vi "check_cancel_token.vi"(8 "error in (no error)":errorcluster) -> (0 "error out":errorcluster, 2 "exit_thread":bool)   [LabVIEW 2021, in "system.threading.lvclass"]
uses:
  system.threading.lvclass
  system.threading.lvclass/system.threading.ctl
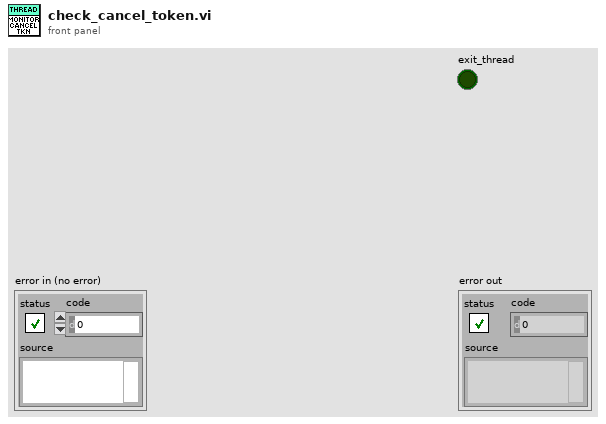
[diagram p1: front panel]
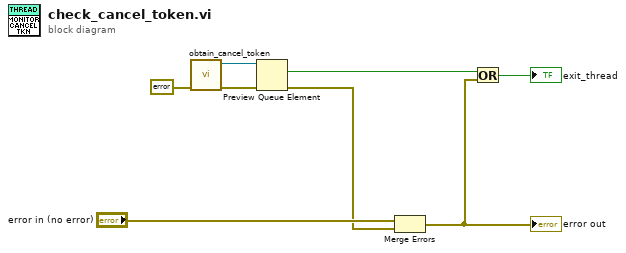
[diagram p0: block diagram]
diagram:
  n1 = call "obtain_cancel_token.vi"("error in (no error)"=errorcluster {"status"=FALSE, "code"=0, "source"=""}) -> ("error out"=w6:errorcluster, "cancel_token"=w7:refnum<queue>)  [unwired: 9 in]
  n2 = Preview Queue Element(queue=w7, error in (no error)=w6) -> (element=w3:bool, error out=w4:errorcluster)  [unwired: 1 in, 2 out]
  n3 = Merge Errors("error in (no error)", w4) -> (w2:errorcluster)
  "error out" <- w2
  n4 = Or(x=w3, y=w2) -> (x .or. y?=→"exit_thread":bool)
